vi "Identify XML Descriptor.vi"(8 "error in":errorcluster, 11 "XML Path in":path) -> (0 "error out":errorcluster, 2 "Found ?":bool, 3 "XML Path out":path, 5 "Custom Device Name":string, 7 "Common Doc Dir":string)   [LabVIEW 2018, in ".LVLIBP CD XML Updater.lvlib" / "Project XML Editor.lvclass"]
uses:
  Project XML Editor.lvclass
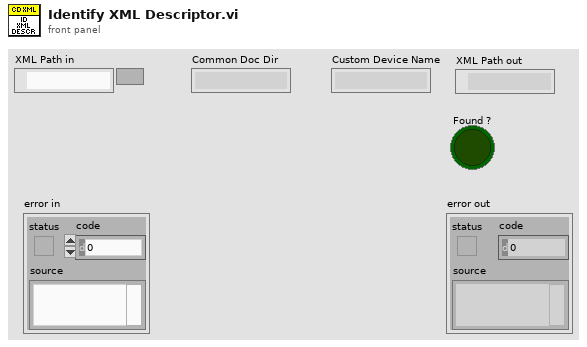
[diagram p1: front panel]
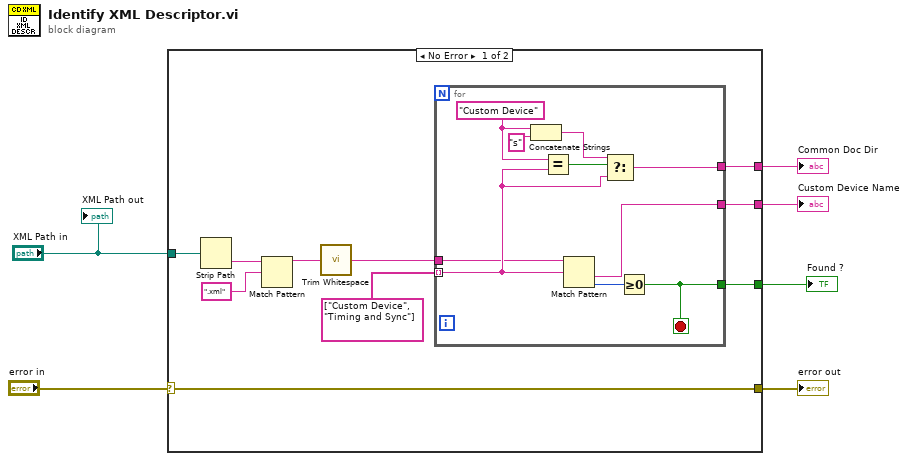
[diagram p0: block diagram]
diagram:
  n1 = case shown="No Error" "error in" {
    selector: "error in" -> [w7 w27]
    tunnel: "XML Path in" -> [w12 _]
    tunnel: [w7 w27] -> w5
    tunnel: [w11 _] -> w4
    tunnel: [w10 _] -> w3
    tunnel: [w8 _] -> w1
    frame No Error {
      n2 = Strip Path(path=w12) -> (name=w9:string)  [unwired: 1 out]
      n3 = Match Pattern(string=w9, regular expression=".xml") -> (before substring=w15:string)  [unwired: 1 in, 3 out]
      n4 = call <vilib>:"Trim Whitespace.vi"("string"=w15) -> ("trimmed string"=w16:string)  [unwired: 1 in]
      n5 = for {
        tunnel: string[] ["Custom Device", "Timing and Sync"] -> [w21] mode=indexing
        tunnel: w16 -> [w18]
        tunnel: [w17] -> w11
        tunnel: [w22] -> w10
        tunnel: [w19] -> w8
        stop <- w19 stop-if-true
        w25 = "Custom Device" ("y")
        n6 = Concatenate Strings(w25, "s" ("string")) -> (w23:string)
        n7 = Equal?(x=w25, y=w21) -> (x = y?=w26:bool)
        n8 = Match Pattern(string=w18, regular expression=w21) -> (after substring=w17:string, offset past match=w20:i32)  [unwired: 1 in, 2 out]
        n9 = Select(t=w23, s=w26, f=w21) -> (s? t:f=w22:string)
        n10 = Greater Or Equal To 0?(x=w20) -> (x >= 0?=w19:bool)
      }
    }
    frame Error {
    }
  }
  "error out" <- w5
  "Found ?" <- w1
  "Custom Device Name" <- w4
  "Common Doc Dir" <- w3
  "XML Path out" <- "XML Path in"
